vi "Add_Ch_to_Block_header.vi"() -> (5 "Plug in titles":string[](array[string]), 7 "Plug in values":string[](array[string]))   [LabVIEW 2010]
uses:
  Globals/Meas_global.vi
  Globals/Plug_in_data_global.vi
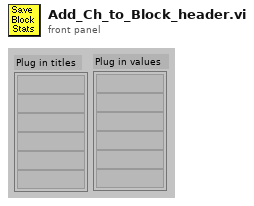
[diagram p1: front panel]
types:
  T1 = typedef "Post_Process.ctl" = enum16{"Take New Data", "Post Process Raw Data File"}
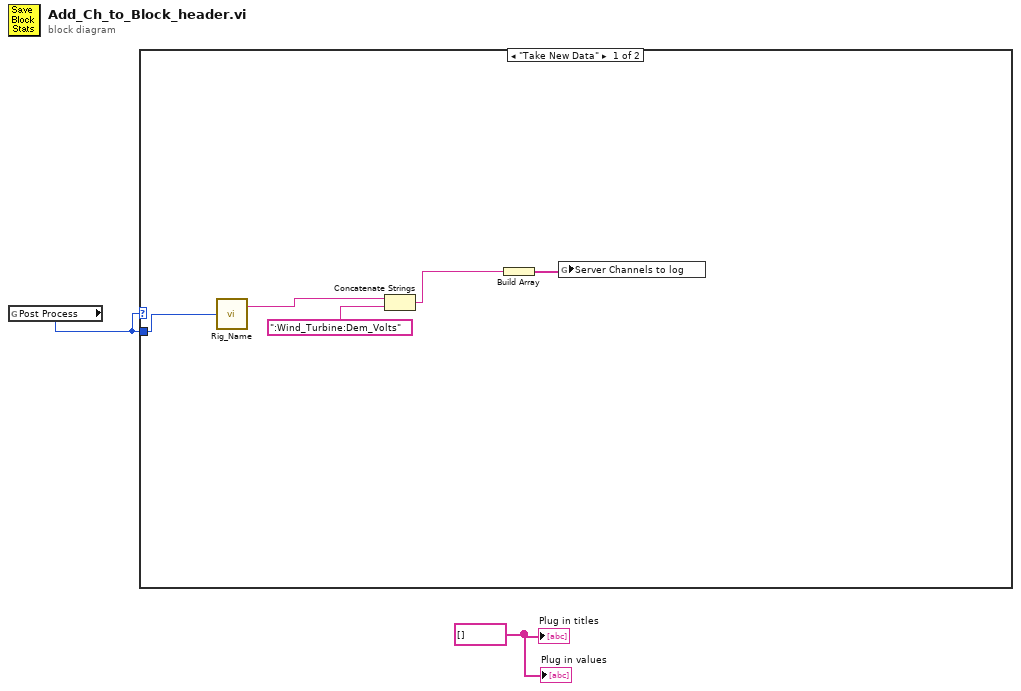
[diagram p0: block diagram]
diagram:
  w2 = string[] [] ("Plug in titles")
  n1 = global read "Meas_global.vi" "Post Process"() -> (w1:T1)
  n2 = case shown="\"Take New Data\"" w1 {
    tunnel: w1 -> [w6 _]
    frame "Take New Data" {
      n3 = call "Rig_Name.vi"("Post Process"=w6) -> ("Rig Setup before dash"=w3:string)  [unwired: 1 out]
      n4 = Concatenate Strings(w3, ":Wind_Turbine:Dem_Volts") -> (w4:string)
      n5 = Build Array(w4) -> (w7:string[])
      n6 = global write "Plug_in_data_global.vi" "Server Channels to log"(w7) -> ()
    }
    frame "Post Process Raw Data File" {
    }
  }
  "Plug in values" <- w2
  "Plug in titles" <- w2
